vi "Init Runtime.vi"(8 "error in (no error)":errorcluster, 10 "data allocations":T1, 11 "Counter Config in":refnum<class "Counter Config.lvclass">) -> (0 "error out":errorcluster, 2 "Skip":bool, 3 "Counter Config out":refnum<class "Counter Config.lvclass">)   [LabVIEW 2015, in "Counter Config.lvclass"]
uses:
  Counter Config.lvclass
  <vilib>/NI/Tag Bus Module Framework/channel/data tables.ctl
  <vilib>/NI/Tag Bus/dictionary/data dictionary.lvclass
  <vilib>/NI/Tag Bus/dictionary table pair.ctl
  <vilib>/NI/Tag Bus/table/data table.ctl
  Counter/Counter.lvclass
  <vilib>/NI/Tag Bus/tag/tag descriptor.lvclass/tag descriptor.ctl
  <vilib>/NI/Tag Bus/tag/read tag name.vi
  <vilib>/NI/Tag Bus/tag/read data type.vi
  <vilib>/NI/Tag Bus/dictionary/locate tag.vi
  <vilib>/NI/Tag Bus Module Framework/channel/TBM channel.lvclass
  <vilib>/NI/Tag Bus/table/data table.lvlib
  <vilib>/NI/Tag Bus/tag bus.lvlib
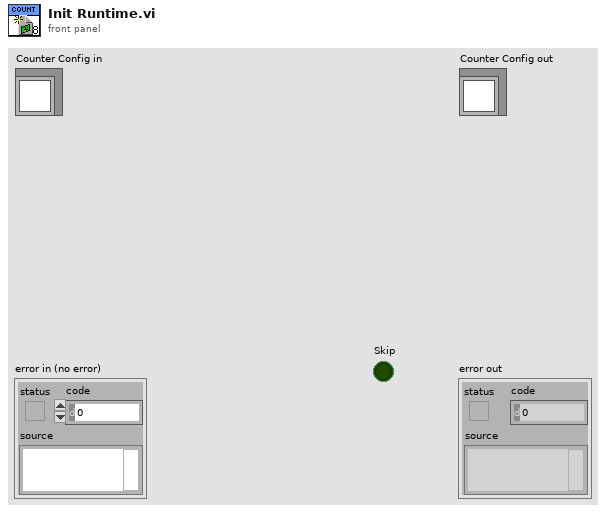
[diagram p1: front panel]
types:
  T1 = typedef "TBM channel.lvclass/data tables.ctl" = cluster{"input data":T2, "processing parameter":T2, "processing result":T2, "output data":T2}
  T2 = typedef "tag bus.lvlib/dictionary table pair.ctl" = cluster{"data dictionary":refnum<class "data dictionary.lvclass">, "data table":T3}
  T3 = typedef "tag bus.lvlib/data table.lvlib/data table.ctl" = cluster{"Double":dbl[], "Single":sgl[], "I64":i64[], "I32":i32[], "I16":i16[], "I8":i8[], "U64":u64[], "U32":u32[], "U16":u16[], "U8":u8[], "Boolean":bool[], "String":string[], "Array of Double":cluster{"DBL Array":dbl[]}[], "Array of Single":cluster{"SGL Array":sgl[]}[], "Array of I64":cluster{"I64 Array":i64[]}[], "Array of I32":cluster{"I32 Array":i32[]}[], "Array of I16":cluster{"I16 Array":i16[]}[], "Array of I8":cluster{"I8 Array":i8[]}[], "Array of U64":cluster{"U64 Array":u64[]}[], "Array of U32":cluster{"U32 Array":u32[]}[], "Array of U16":cluster{"U16 Array":u16[]}[], "Array of U8":cluster{"U8 Array":u8[]}[], "Array of Boolean":cluster{"Boolean Array":bool[]}[], "Array of String":cluster{"String Array":string[]}[]}
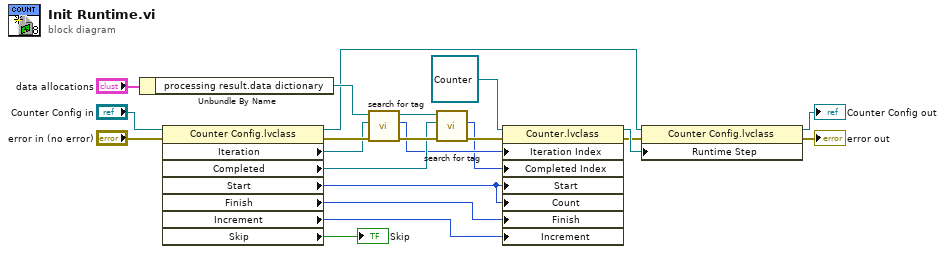
[diagram p0: block diagram]
diagram:
  n1 = Unbundle By Name("data allocations") -> ("processing result.data dictionary"=w16:refnum<class "data dictionary.lvclass">)
  n2 = property class="Counter Config.lvclass"(reference="Counter Config in", error in="error in (no error)") -> (reference out=w14:refnum<class "Counter Config.lvclass">, error out=w7:errorcluster, "Iteration"=w5:refnum<class "TBM channel.lvclass">, "Completed"=w4:refnum<class "TBM channel.lvclass">, "Start"=w1:i32, "Finish"=w19:i32, "Increment"=w18:i32, "Skip"=→"Skip":bool)
  n3 = call <vilib>:"search for tag.vi"("error in"=w7, "system tag"=w5, "data dictionary in"=w16) -> ("error out"=w9:errorcluster, "index"=w3:i32, "data dictionary out"=w15:refnum<class "data dictionary.lvclass">)  [unwired: 6 in]
  n4 = call <vilib>:"search for tag.vi"("error in"=w9, "system tag"=w4, "data dictionary in"=w15) -> ("error out"=w8:errorcluster, "index"=w2:i32)  [unwired: 6 in, 1 out]
  n5 = property class="Counter.lvclass"(reference=refnum<class "Counter.lvclass"> refnum ("Counter.lvclass"), error in=w8, "Iteration Index"=w3, "Completed Index"=w2, "Start"=w1, "Count"=w1, "Finish"=w19, "Increment"=w18) -> (reference out=w13:refnum<class "Counter.lvclass">, error out=w10:errorcluster)
  n6 = property class="Counter Config.lvclass"(reference=w14, error in=w10, "Runtime Step"=w13) -> (reference out=→"Counter Config out":refnum<class "Counter Config.lvclass">, error out=→"error out":errorcluster)
